vi "LV2GSettings.vi"(7 "Operation":T2, 8 "error in (no error)":errorcluster, 11 "Settings":T1={"DMM Settings"={"Port"="", "baud rate"=9600, "data bits"=8, "stop bits"=10, "parity"=enum."None", "flow control"=enum."None"}, "Modbus Settings"={"Port"="", "baud rate"=9600, "parity"=enum."None", "flow control"=enum."None"}} {"DMM Settings"."data bits" min=5 max=8 step=1}) -> (0 "error out":errorcluster, 3 "Settings out":T1={"DMM Settings"={"Port"="", "baud rate"=9600, "data bits"=8, "stop bits"=10, "parity"=enum."None", "flow control"=enum."None"}, "Modbus Settings"={"Port"="", "baud rate"=9600, "parity"=enum."None", "flow control"=enum."None"}} {"DMM Settings"."data bits" min=5 max=8 step=1})   [LabVIEW 2011]
uses:
  Strict Type Controls/Settings Operation.ctl
  Strict Type Controls/Settings.ctl
  <vilib>/Utility/config.llb/NI_LVConfig.lvlib
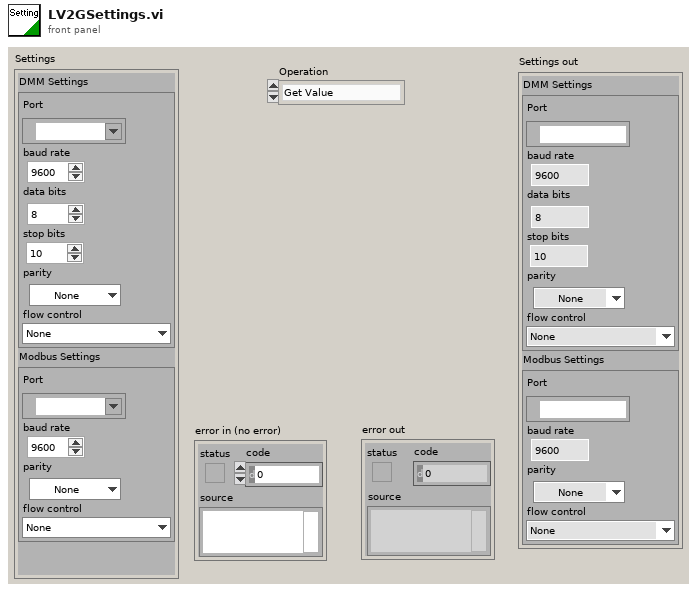
[diagram p1: front panel]
types:
  T1 = typedef "Settings.ctl" = cluster{"DMM Settings":cluster{"Port":refnum<visa-resource-name>, "baud rate":u32, "data bits":u16, "stop bits":u16, "parity":enum16{"None", "Odd", "Even", "Mark", "Space"}, "flow control":enum16{"None", "XON/XOFF", "RTS/CTS", "XON/XOFF & RTS/CTS", "DTR/DSR", "XON/XOFF & DTR/DSR"}}, "Modbus Settings":cluster{"Port":refnum<visa-resource-name>, "baud rate":u32, "parity":enum16{"None", "Odd", "Even", "Mark", "Space"}, "flow control":enum16{"None", "XON/XOFF", "RTS/CTS", "XON/XOFF & RTS/CTS", "DTR/DSR", "XON/XOFF & DTR/DSR"}}}
  T2 = typedef "Settings Operation.ctl" = enum8{"Get Value", "Set Value", "Read File", "Write File", "Write Stored Value"}
  T3 = typedef "NI_LVConfig.lvlib/Config Data RefNum.ctl" = refnum<k1>
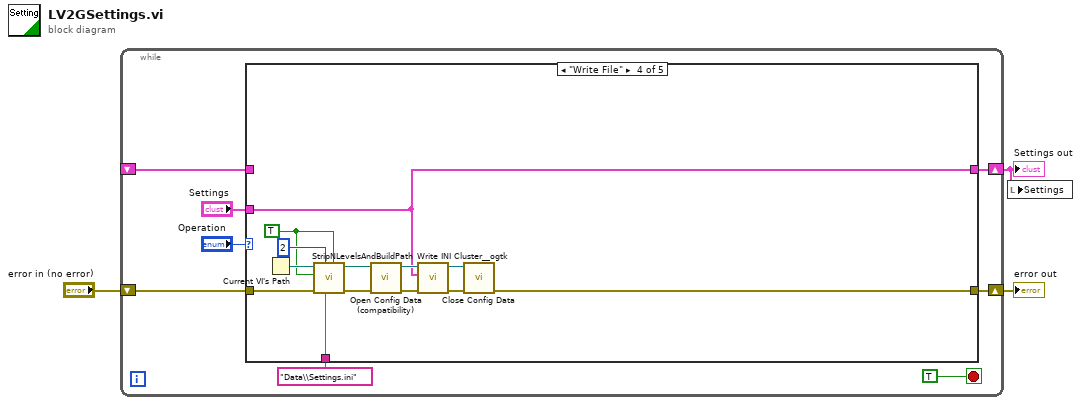
[diagram p0: block diagram]
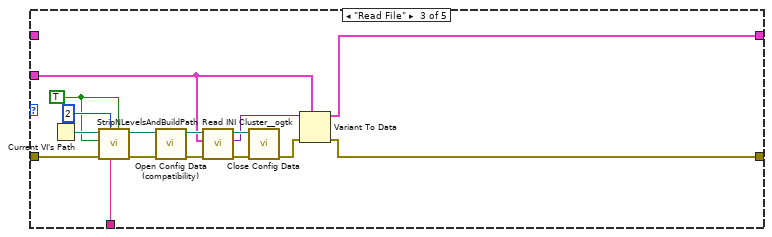
[diagram p4: hidden frame]
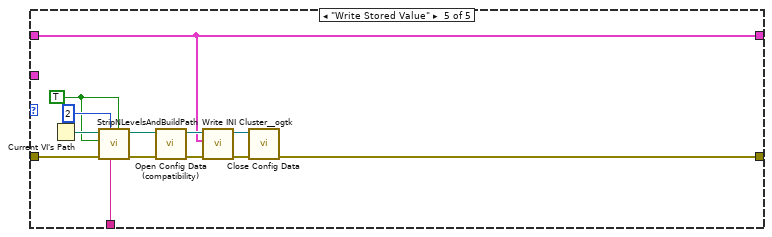
[diagram p5: hidden frame]
diagram:
  n1 = while {
    shift-right: [w10] -> w2
    shift-left: _ -> [w11]
    shift-right: [w7] -> w1
    shift-left: "error in (no error)" -> [w8]
    stop <- TRUE stop-if-true
    n2 = case shown="\"Write File\"" "Operation" {
      tunnel: w11 -> [w13 _ _ _ w46]
      tunnel: [w13 w15 w19 w33 w46] -> w10
      tunnel: "Settings" -> [_ w15 w20 w33 _]
      tunnel: w8 -> [w12 w14 w22 w43 w48]
      tunnel: [w12 w14 w16 w34 w47] -> w7
      tunnel: "Data\\Settings.ini" ("Build Path") -> [_ _ w17 w32 w45]
      frame "Get Value" {
      }
      frame "Set Value" {
      }
      frame "Read File" {
        w29 = TRUE ("Is File?")
        n3 = Current VI's Path() -> (path=w31:path)
        n4 = call "StripNLevelsAndBuildPath.vi"("Create Folders"=w29, "Build Path"=w17, "Strip Levels"=2, "error in(no error)"=w22, "Is File"=w29, "Path In"=w31) -> ("error out"=w23:errorcluster, "Path Out"=w28:path)  [unwired: 4 out]
        n5 = call <vilib>:"Open Config Data (compatibility).vi"("error in (no error)"=w23, "configuration file path"=w28) -> ("error out"=w26:errorcluster, "refnum"=w27:T3)  [unwired: 7 in, 1 out]
        n6 = call <userlib>:"Read INI Cluster__ogtk.vi"("error in (no error)"=w26, "INI Fomatted Cluster Type"=w20, "refnum"=w27) -> ("error out"=w25:errorcluster, "INI Fomatted Cluster"=w21:variant, "dup refnum"=w24:T3)  [unwired: 6 out]
        n7 = call <vilib>:"Close Config Data.vi"("error in (no error)"=w25, "refnum"=w24) -> ("error out"=w18:errorcluster)  [unwired: 1 in, 8 out]
        n8 = Variant To Data(error in=w18, type=w20, Variant=w21) -> (data=w19:T1, error out=w16:errorcluster)
      }
      frame "Write File" {
        w41 = TRUE ("Is File?")
        n9 = Current VI's Path() -> (path=w44:path)
        n10 = call "StripNLevelsAndBuildPath.vi"("Create Folders"=w41, "Build Path"=w32, "Strip Levels"=2, "error in(no error)"=w43, "Is File"=w41, "Path In"=w44) -> ("error out"=w35:errorcluster, "Path Out"=w40:path)  [unwired: 4 out]
        n11 = call <vilib>:"Open Config Data (compatibility).vi"("error in (no error)"=w35, "configuration file path"=w40) -> ("error out"=w38:errorcluster, "refnum"=w39:T3)  [unwired: 7 in, 1 out]
        n12 = call <userlib>:"Write INI Cluster__ogtk.vi"("error in (no error)"=w38, "INI Fomatted Cluster"=w33, "refnum"=w39) -> ("error out"=w37:errorcluster, "dup refnum"=w36:T3)  [unwired: 1 in, 6 out]
        n13 = call <vilib>:"Close Config Data.vi"("error in (no error)"=w37, "refnum"=w36) -> ("error out"=w34:errorcluster)  [unwired: 1 in, 8 out]
      }
      frame "Write Stored Value" {
        w55 = TRUE ("Is File?")
        n14 = Current VI's Path() -> (path=w57:path)
        n15 = call "StripNLevelsAndBuildPath.vi"("Create Folders"=w55, "Build Path"=w45, "Strip Levels"=2, "error in(no error)"=w48, "Is File"=w55, "Path In"=w57) -> ("error out"=w49:errorcluster, "Path Out"=w54:path)  [unwired: 4 out]
        n16 = call <vilib>:"Open Config Data (compatibility).vi"("error in (no error)"=w49, "configuration file path"=w54) -> ("error out"=w52:errorcluster, "refnum"=w53:T3)  [unwired: 7 in, 1 out]
        n17 = call <userlib>:"Write INI Cluster__ogtk.vi"("error in (no error)"=w52, "INI Fomatted Cluster"=w46, "refnum"=w53) -> ("error out"=w51:errorcluster, "dup refnum"=w50:T3)  [unwired: 1 in, 6 out]
        n18 = call <vilib>:"Close Config Data.vi"("error in (no error)"=w51, "refnum"=w50) -> ("error out"=w47:errorcluster)  [unwired: 1 in, 8 out]
      }
    }
  }
  "error out" <- w1
  "Settings out" <- w2
  n19 = local write "Settings"(w2) -> ()
